vi "Get DDS Trigger Source Io.vi"(11 "channel_index":u8) -> (3 "function return":u32)   [LabVIEW 2021, in "vmmso.lvlib"]
doc: "DLL_API unsigned int WINAPI GetDDSTriggerSourceIo(unsigned char channel_index);"
uses:
  vmmso.lvlib
  vmmso.dll
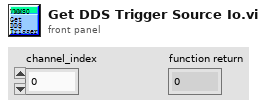
[diagram p1: front panel]
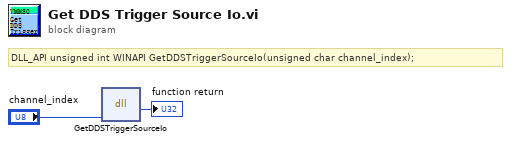
[diagram p0: block diagram]
diagram:
  # "DLL_API unsigned int WINAPI GetDDSTriggerSourceIo(unsigned char channel_index);"
  n1 = dll-call lib="D:/labviewdemo/LabviewDemo 21/vmmso/vmmso.*" fn="GetDDSTriggerSourceIo"("channel_index"="channel_index") -> (→"function return":u32)  [unwired: 4 in, 2 out]
